vi "Init FPGA.vi"(8 "error in (no error)":errorcluster, 10 "Controller Config":T1, 11 "FPGA Ref":T3) -> (0 "error out":errorcluster, 3 "FPGA Ref Out":T3)   [LabVIEW 2013]
uses:
  Controls/FPGA_Reference.ctl
  Controls/Controller Config.ctl
  Type Defs/Controller Names.ctl
  <vilib>/FPGAPlugInAG/sbRIO-9626/niLvFpga_Reset_sbRIO-9626.vi
  <vilib>/Utility/error.llb/Error Cluster From Error Code.vi
  <vilib>/rvi/errors/niLvFpgaAdjustHostInterfaceError.vi
  <vilib>/FPGAPlugInAG/sbRIO-9626/niLvFpga_Run_sbRIO-9626.vi
  <vilib>/rvi/interface/nirviMethod/nirviMethod.xnode
  FPGA/bitfiles/TI sbRIO PWM (FPGA) v1.0.lvbitx
  <vilib>/rvi/interface/nirviReadWriteControl/nirviReadWriteControl.xnode
  <userlib>/_NI SPI IP/FPGA/Controllers/Public/Transfer Settings.ctl
  <userlib>/_NI SPI IP/FPGA/Controllers/DIO SPI FPGA.lvlib
  NiFpgaLv.dll
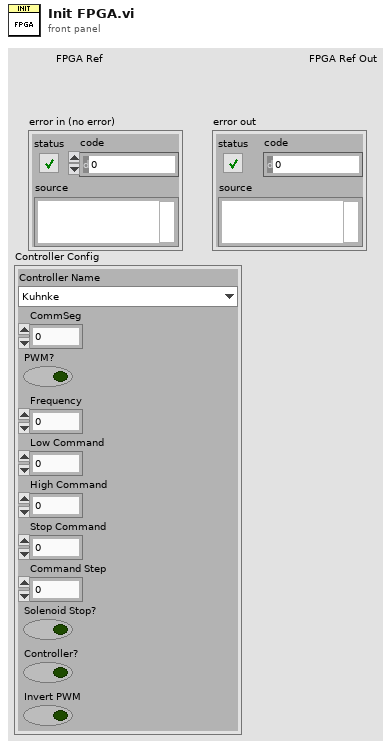
[diagram p1: front panel]
types:
  T1 = typedef "Controller Config.ctl" = cluster{"Controller Name":T2, "CommSeg":i32, "PWM?":bool, "Frequency":i32, "Low Command":dbl, "High Command":dbl, "Stop Command":dbl, "Command Step":dbl, "Solenoid Stop?":bool, "Controller?":bool, "Invert PWM":bool}
  T2 = typedef "Controller Names.ctl" = enum16{"Kuhnke", "Helbako BLDC", "Conti", "Hella BLDC OL PWM", "Hella BLDC Turbine OL PWM", "Hella BLDC Pressure", "Helbako (old)", "TI PWM", "PSA", "Hella Gas", "Hella Diesel", "8 Comm", "10 Comm", "8 Comm Hella", "10 Comm Hella", "8 Comm Omron", "10 Comm Omron", "8 Comm Nissan", "10 Comm Nissan"}
  T3 = typedef "FPGA_Reference.ctl" = refnum<k20>
  T4 = cluster{"Divide Value":u8, "Transfer Length (bits)":u8, "CS Asserted Polarity":bool, "Clock Polarity (CPOL)":bool, "Clock Phase (CPHA)":bool, "Lengthen MISO Setup":bool, "Direction Change Bit":u8, "MOSI Starts as Output":bool, "Tristatable MOSI":bool}
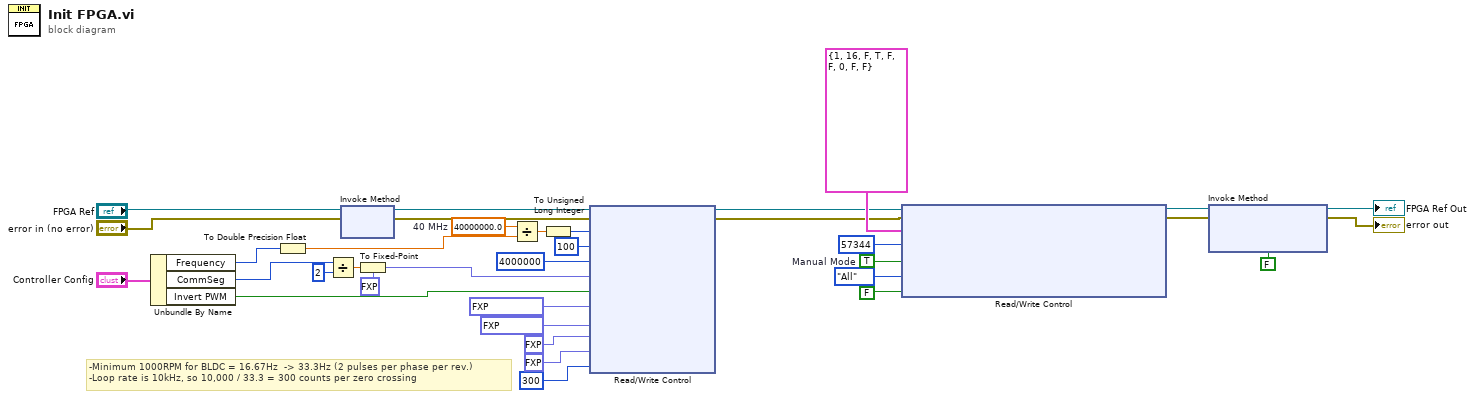
[diagram p0: block diagram]
diagram:
  w22 = 40000000.0  # 40 MHz
  w32 = TRUE  # Manual Mode
  # "-Minimum 1000RPM for BLDC = 16.67Hz  -> 33.3Hz (2 pulses per phase per rev.)\n-Loop rate is 10kHz, so 10,000 / 33.3 = 300 counts per zero crossing"
  n1 = Unbundle By Name("Controller Config") -> ("Frequency"=w7:i32, "CommSeg"=w9:i32, "Invert PWM"=w8:bool)
  n2 = To Double Precision Float(number=w7) -> (double precision float=w6:dbl)
  n3 = Divide(x=w9, y=2) -> (x/y=w17:dbl)
  n4 = xnode "Invoke Method"("FPGA VI Reference In"="FPGA Ref", "error in"="error in (no error)") -> ("FPGA VI Reference Out"=w21:T3, "error out"=w26:errorcluster)
  n5 = To Fixed-Point(fixed-point type=fxp<+,32,16> 0.0 ("CommFactor"), number=w17) -> (fixed-point=w27:fxp<+,32,16>)
  n6 = Divide(x=w22, y=w6) -> (x/y=w25:dbl)
  n7 = To Unsigned Long Integer(number=w25) -> (unsigned 32bit integer=w24:u32)
  n8 = xnode "Read/Write Control"("FPGA VI Reference In"=w21, "error in"=w26, "PWM Period (Ticks)"=w24, "Loop Timer (uSec)"=u32 100, "AI Divisor"=u32 4000000 ("x"), "CommFactor"=w27, "InvertPWM?"=w8, "PumpCurrentB"=fxp<+/-,16,9> -121.7265625, "PumpCurrentM"=fxp<+/-,16,9> 74.5546875, "Speed Thshld"=fxp<+/-,24,7> -1.0, "Current Threshold"=fxp<+,26,7> 2.0, "Speed Timout (cnts)"=u64 300) -> ("FPGA VI Reference Out"=w13:T3, "error out"=w12:errorcluster)
  n9 = xnode "Read/Write Control"("FPGA VI Reference In"=w13, "error in"=w12, "ADC SPI Settings"=T4 {"Divide Value"=1, "Transfer Length (bits)"=16, "CS Asserted Polarity"=FALSE, "Clock Polarity (CPOL)"=TRUE, "Clock Phase (CPHA)"=FALSE, "Lengthen MISO Setup"=FALSE, "Direction Change Bit"=0, "MOSI Starts as Output"=FALSE, "Tristatable MOSI"=FALSE} ("Master Settings"), "ADC Data In"=u64 57344 ("data to write"), "ADC Manual"=w32, "ADC CS Mode"=enum16{"All", "CS0", "CS1"}."All" ("Mode"), "ADC Trigger"=FALSE ("nx-100 Trigger")) -> ("FPGA VI Reference Out"=w4:T3, "error out"=w3:errorcluster)
  n10 = xnode "Invoke Method"("FPGA VI Reference In"=w4, "error in"=w3, "Wait Until Done (F)"=FALSE) -> ("FPGA VI Reference Out"=→"FPGA Ref Out":T3, "error out"=→"error out":errorcluster)
